vi "Variant to Class.vi"(8 "error in (no error)":errorcluster, 10 "Data in":variant, 11 "Build Job in":refnum<class "Build Job.lvclass">) -> (0 "error out":errorcluster, 2 "Data Out":variant, 3 "Build Job out":refnum<class "Build Job.lvclass">)   [LabVIEW 2014, in "Build Job.lvclass"]
uses:
  Build Job.lvclass
  Build Job.lvclass/Build Job.ctl
  Serializable Node/Serializable Node.lvclass
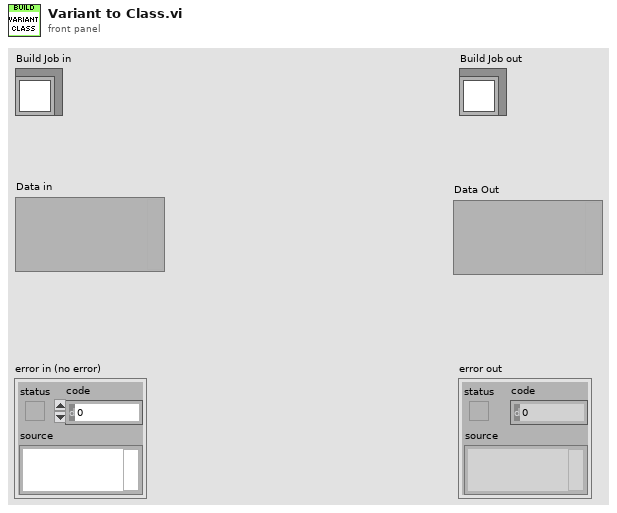
[diagram p1: front panel]
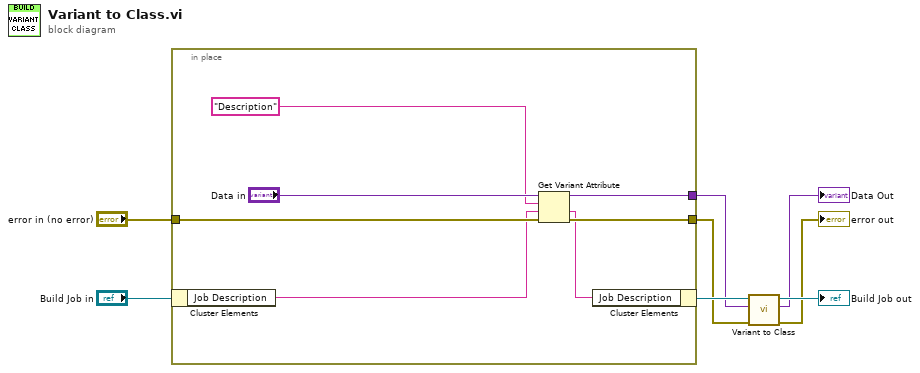
[diagram p0: block diagram]
diagram:
  n1 = in-place {
    in-place-border: "error in (no error)" -> [w14]
    in-place-border: [w13] -> w1
    in-place-border: [w12] -> w3
    n2 = in-place-cluster #1("Build Job in") -> ("Job Description"=w10:string)
    n3 = Get Variant Attribute(Variant="Data in", name="Description", default value (empty Variant)=w10, error in=w14) -> (duplicate Variant=w12:variant, value=w9:string, error out=w13:errorcluster)  [unwired: 1 out]
    n4 = in-place-cluster #1("Job Description"=w9) -> (w6:refnum<class "Build Job.lvclass">)
  }
  n5 = call-parent "Variant to Class.vi"("error in (no error)"=w1, "Data in"=w3, "Serializable Node in"=w6) -> ("error out"=→"error out":errorcluster, "Data Out"=→"Data Out":variant, "Serializable Node out"=→"Build Job out":refnum<class "Build Job.lvclass">)  [unwired: 6 in]
